vi "Time.vi"(8 "error in (no error)":errorcluster, 10 "Control In":T1, 11 "CAD Dispense in":refnum<class "CAD Dispense.lvclass">) -> (0 "error out":errorcluster, 1 "Timing Data":i32[](array[numeric]), 2 "Control Out":T1, 3 "CAD Dispense out":refnum<class "CAD Dispense.lvclass">)   [LabVIEW 2019, in "CAD Dispense.lvclass"]
uses:
  CAD Dispense.lvclass
  Controller/Controllers.ctl
  Controller/I-O/I-O.lvclass
  Controller/Dispenser/Dispenser.lvclass
  C:/Program Files (x86)/Aerotech/A3200/LabVIEW/2010/Bin/Aerotech.A3200.dll
  Program Files (x86)/Aerotech/A3200/LabVIEW/2010/Bin/Aerotech.A3200.dll
  CAD Dispense.lvclass/CAD Dispense.ctl
  Controller/Motion/A3200/A3200.lvclass
  Controller/Controller.lvclass
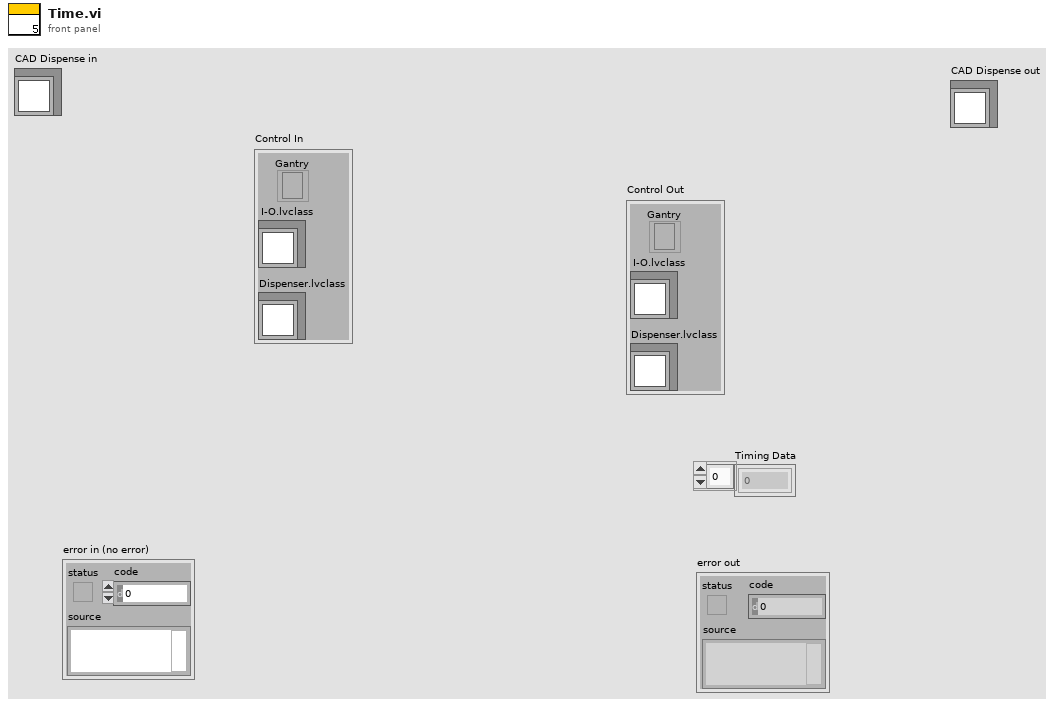
[diagram p1: front panel]
types:
  T1 = typedef "Controller.lvclass/Controllers.ctl" = cluster{"I-O.lvclass":refnum<class "I-O.lvclass">, "Dispenser.lvclass":refnum<class "Dispenser.lvclass">, "Gantry":refnum<k24>}
  T2 = cluster{"Motion":dbl[][], "Center":dbl[], "Circle?":bool, "CW/CCW":dbl}[]
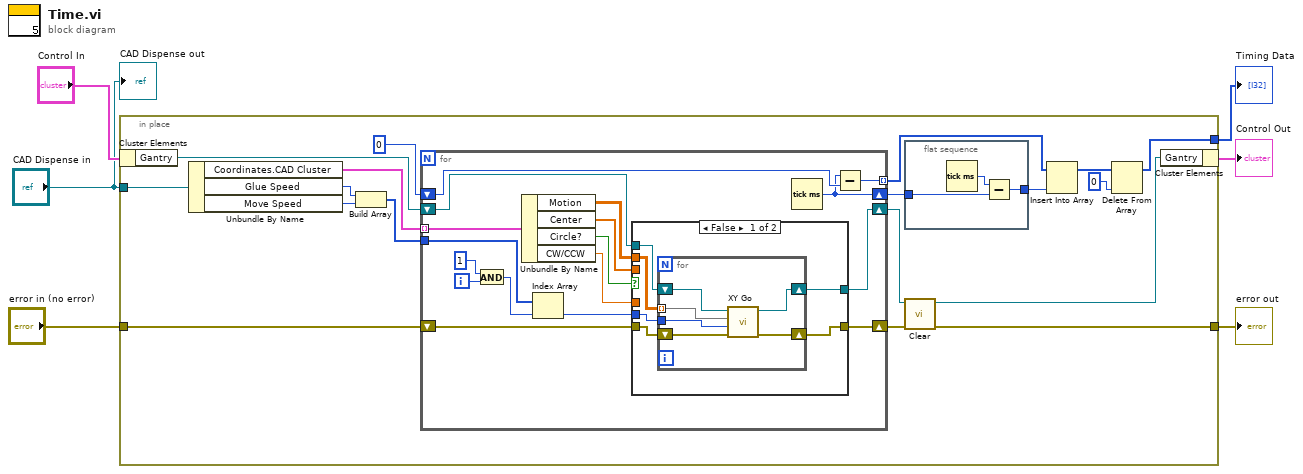
[diagram p0: block diagram]
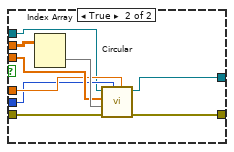
[diagram p2: hidden frame]
diagram:
  n1 = in-place {
    in-place-border: "CAD Dispense in" -> [w24]
    in-place-border: [w13] -> w3
    in-place-border: "error in (no error)" -> [w9]
    in-place-border: [w7] -> w1
    n2 = in-place-cluster #1("Control In") -> ("Gantry"=w12:refnum<k24>)
    n3 = Unbundle By Name(w24) -> ("Coordinates.CAD Cluster"=w14:T2, "Glue Speed"=w16:i32, "Move Speed"=w15:i32)
    n4 = Build Array(w16, w15) -> (w17:i32[])
    n5 = for {
      shift-right: [w39] -> w18
      shift-left: u32 0 ("millisecond timer value") -> [w42]
      tunnel: [w41] -> w20 mode=indexing
      tunnel: w14 -> [w37] mode=indexing
      tunnel: w17 -> [w33]
      shift-right: [w30] -> w11
      shift-left: w12 -> [w31]
      shift-right: [w28] -> w8
      shift-left: w9 -> [w29]
      i -> [w43]
      n6 = And(x=1, y=w43) -> (x .and. y?=w40:i32)
      n7 = Unbundle By Name(w37) -> ("Motion"=w36:dbl[][], "Center"=w35:dbl[], "Circle?"=w34:bool, "CW/CCW"=w32:dbl)
      n8 = Index Array(array=w33, index=w40) -> (element=w38:i32)
      n9 = case shown="False" w34 {
        tunnel: w38 -> [w50 w61]
        tunnel: [w47 w59] -> w30
        tunnel: w36 -> [w48 w65]
        tunnel: w35 -> [_ w63]
        tunnel: w32 -> [_ w62]
        tunnel: w31 -> [w49 w60]
        tunnel: w29 -> [w46 w58]
        tunnel: [w45 w57] -> w28
        frame False {
          n10 = for {
            tunnel: w50 -> [w53]
            tunnel: w48 -> [w54] mode=indexing
            shift-right: [w56] -> w47
            shift-left: w49 -> [w55]
            shift-right: [w51] -> w45
            shift-left: w46 -> [w52]
            n11 = call "XY Go.vi"("error in (no error)"=w52, "Speed"=w53, "XY"=w54, "Gantry In"=w55) -> ("error out"=w51:errorcluster, "Gantry Out"=w56:refnum<k24>)  [unwired: 6 in]
          }
        }
        frame True {
          n12 = Index Array(array=w65) -> (element=w64:dbl[])  [unwired: 2 in]
          n13 = call "Circular.vi"("Direction"=w62, "Speed"=w61, "error in (no error)"=w58, "XY End"=w64, "XY Center"=w63, "Gantry In"=w60) -> ("error out"=w57:errorcluster, "Gantry Out"=w59:refnum<k24>)  [unwired: 4 in]
        }
      }
      n14 = Tick Count (ms)() -> (millisecond timer value=w39:u32)
      n15 = Subtract(x=w39, y=w42) -> (x-y=w41:u32)
    }
    n16 = flat-sequence {
      tunnel: [w26] -> w21
      tunnel: w18 -> [w25]
      frame #0 {
        n17 = Tick Count (ms)() -> (millisecond timer value=w27:u32)
        n18 = Subtract(x=w27, y=w25) -> (x-y=w26:u32)
      }
    }
    n19 = call "Clear.vi"("error in (no error)"=w8, "Gantry In"=w11) -> ("error out"=w7:errorcluster, "Gantry Out"=w10:refnum<k24>)  [unwired: 8 in]
    n20 = Insert Into Array(array=w20, new element=w21) -> (w19:u32[])  [unwired: 1 in]
    n21 = Delete From Array(array=w19, index=0) -> (array with subset deleted=w13:u32[])  [unwired: 1 in, 1 out]
    n22 = in-place-cluster #1("Gantry"=w10) -> (→"Control Out":T1)
  }
  "error out" <- w1
  "Timing Data" <- w3
  "CAD Dispense out" <- "CAD Dispense in"
